vi "resave_camera_images_parfor.vi"() -> ()   [LabVIEW 2019]
uses:
  <vilib>/vision/NI_Vision_Development_Module.lvlib
panel:
  out "Display Array":i32[](array[numeric])
  out "Processed Frames/s":dbl
  out "error out":errorcluster
  in  "Experiment Folder In":string="C:\\Data\\20200217_HeadTailContinuousGWN_test\\Data20200217_115033\\"
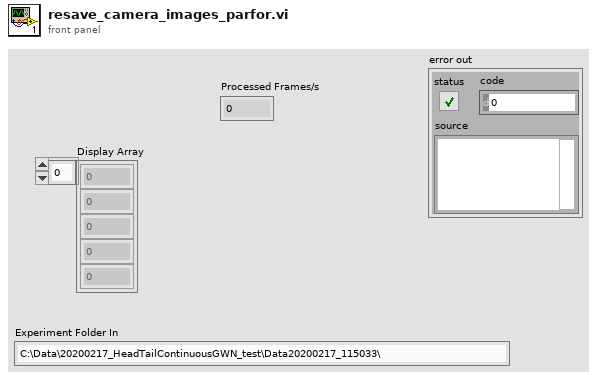
[diagram p1: front panel]
types:
  T1 = typedef "Image Type" = u32
  T2 = typedef "IMAQ Image.ctl" = refnum<image>
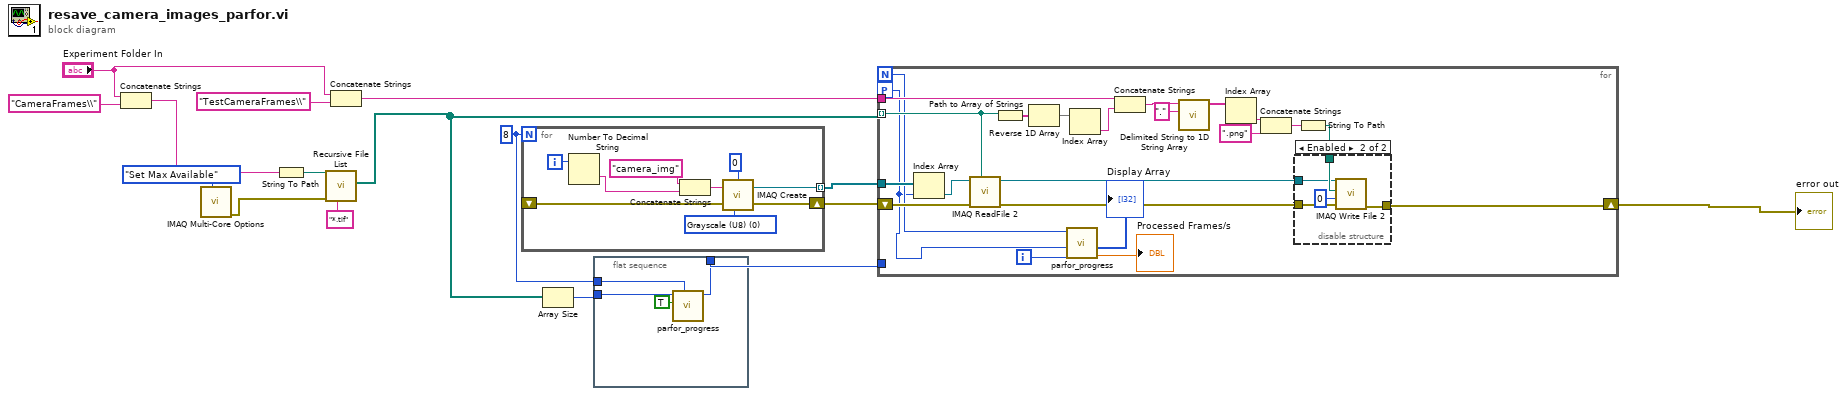
[diagram p0: block diagram]
diagram:
  w1 = 8
  n1 = Concatenate Strings("Experiment Folder In", "CameraFrames\\" ("string")) -> (w15:string)
  n2 = call "IMAQ Multi-Core Options"("Get/Set Number of Cores (Get)"=enum32{"Get", "Set", "Set Max Available"}."Set Max Available") -> ("error out"=w9:errorcluster)  [unwired: 9 in, 1 out]
  n3 = String To Path(string=w15) -> (path=w13:path)
  n4 = call <vilib>:"Recursive File List.vi"("pattern"="*.tif", "error in (no error)"=w9, "Folder Path"=w13) -> ("All Files in Dir"=w3:path[])  [unwired: 4 in, 4 out]
  n5 = Concatenate Strings("Experiment Folder In", "TestCameraFrames\\" ("string")) -> (w8:string)
  n6 = for {
    N: w1 -> [_]
    shift-right: [w18] -> w7
    shift-left: _ -> [w20]
    tunnel: [w22] -> w6 mode=indexing
    i -> [w25]
    w17 = T1 0 items=["Grayscale (U8)", "Grayscale (I16)", "Grayscale (SGL)", "Complex (CSG)", "RGB (U32)", "HSL (U32)", "RGB (U64)", "Grayscale (U16)"] ("Image Type")
    n7 = Number To Decimal String(number=w25) -> (decimal integer string=w21:string)  [unwired: 1 in]
    n8 = Concatenate Strings("camera_img", w21) -> (w24:string)
    n9 = call "IMAQ Create"("Border Size"=0, "Image Name"=w24, "Image Type"=w17, "error in (no error)"=w20) -> ("New Image"=w22:T2, "error out"=w18:errorcluster)  [unwired: 1 in]
  }
  n10 = Array Size(array=w3) -> (size(s)=w2:i32)
  n11 = flat-sequence {
    tunnel: [w28] -> w4
    tunnel: w2 -> [w27]
    tunnel: w1 -> [w26]
    frame #0 {
      n12 = call "parfor_progress.vi"("Parpool Count"=w26, "reset"=TRUE, "N"=w27) -> ("Percent Count"=w28:i32)  [unwired: 6 in, 2 out]
    }
  }
  n13 = for {
    N -> [w33]
    tunnel: w3 -> [w47] mode=indexing
    tunnel: w6 -> [w36]
    tunnel: w8 -> [w46]
    shift-right: [w43] -> w5
    shift-left: w7 -> [w52]
    workers-P: _ -> [w32]
    tunnel: w4 -> [_]
    i -> [w31]
    n14 = Index Array(array=w36, index=w32) -> (element=w35:T2)
    n15 = call "IMAQ ReadFile 2"("File Path"=w47, "error in (no error)"=w52, "Image"=w35) -> ("error out"=w51:errorcluster, "Image Out"=w50:T2)  [unwired: 4 in, 3 out]
    n16 = Path to Array of Strings(0:w47) -> (2:w49:string[])  [unwired: 1 out]
    n17 = Reverse 1D Array(array=w49) -> (reversed array=w48:string[])
    n18 = call "parfor_progress.vi"("Current Display"=w31, "PID"=w32, "N"=w33) -> ("Processing Rate"=→"Processed Frames/s":dbl, "Display Array"=→"Display Array":i32[])  [unwired: 6 in, 1 out]
    n19 = Index Array(array=w48) -> (element=w45:string)  [unwired: 1 in]
    n20 = Concatenate Strings(w46, w45) -> (w42:string)
    n21 = call <vilib>:"Delimited String to 1D String Array.vi"("delimiter"=".", "delimited string"=w42) -> ("string array"=w40:string[])  [unwired: 9 in]
    n22 = Index Array(array=w40) -> (element=w39:string)  [unwired: 1 in]
    n23 = Concatenate Strings(w39, ".png" ("string")) -> (w37:string)
    n24 = String To Path(string=w37) -> (path=w44:path)
    n25 = disable-structure shown="Enabled" {
      disable-tunnel: w51 -> [_ w57]
      disable-tunnel: w50 -> [_ w54]
      disable-tunnel: w44 -> [_ w55]
      disable-tunnel: [_ w56] -> w43
      frame Disabled {
      }
      frame Enabled {
        n26 = call-poly "IMAQ Write File 2"("error in (no error)"=w57, "Image Quality"=u32 0, "File Path"=w55, "Image"=w54) -> ("error out"=w56:errorcluster)  [unwired: 6 in, 1 out]
      }
    }
  }
  "error out" <- w5
